vi "image.vi"(0 "Camera in":refnum<class "Camera.lvclass">, 5 "data_format":T2(ring)=enum."Mono16", 7 "image_index":u32, 9 "roi":cluster{"x0":u64, "y0":u64, "x1":u64, "y1":u64}={"x0"=18446744073709551615, "y0"=18446744073709551615, "x1"=18446744073709551615, "y1"=18446744073709551615}, 11 "error in (no error)":errorcluster, 12 "PCO_Recorder_CompressionParams":T5={"dGainK"=nan, "dDarkNoise_e"=nan, "dDSNU_e"=nan, "dPRNU_pct"=nan, "dLightSourceNoise_pct"=0.0}) -> (2 "timestamp":T4 {"lvTimestamp" format="%<%.6X\n%x>T"}, 3 "meta_data":T3, 4 "Camera out":refnum<class "Camera.lvclass">, 6 "image (U8)":u8[][](array[numeric]), 8 "image (U32)":u32[][](array[numeric]), 10 "image (U64)":T1(array[cluster]), 14 "raw_image (U16)":u16[][](array[numeric]), 15 "error out":errorcluster)   [LabVIEW 2019, in "Camera.lvclass"]
doc: "Get an image from the recorder. The type of the image is 2D array of pixel values. This array is\nshaped depending on the resolution and ROI of the image."
uses:
  Camera.lvclass
  pco.recorder/Recorder.lvlib
  pco.convert/Convert.lvlib
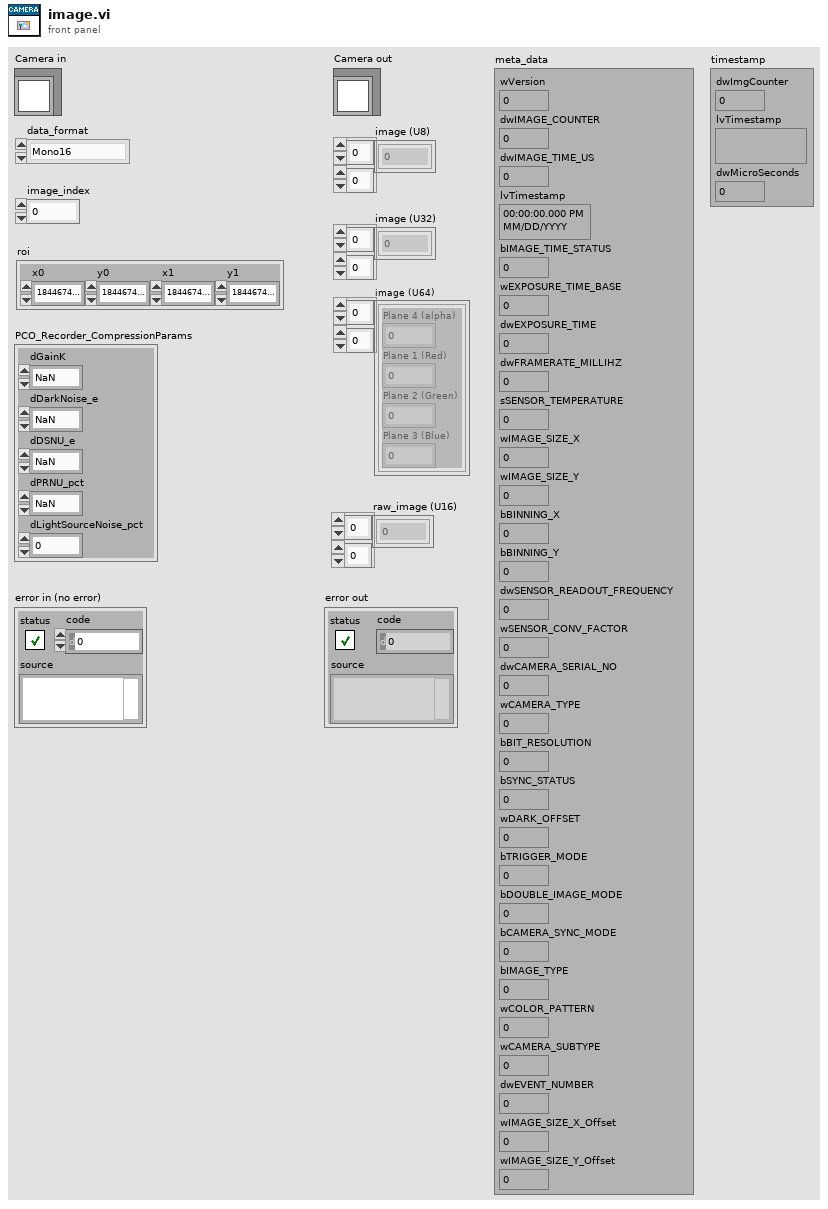
[diagram p1: front panel]
types:
  T1 = cluster{"Plane 4 (alpha)":u16, "Plane 1 (Red)":u16, "Plane 2 (Green)":u16, "Plane 3 (Blue)":u16}[][]
  T2 = enum16{"Undefined", "Mono8", "Mono16", "BGRA8", "RGBA8", "BGRA16", "RGBA16", "CompressedMono8"}
  T3 = cluster{"wVersion":u16, "dwIMAGE_COUNTER":u32, "dwIMAGE_TIME_US":u32, "lvTimestamp":timestamp, "bIMAGE_TIME_STATUS":u8, "wEXPOSURE_TIME_BASE":u16, "dwEXPOSURE_TIME":u32, "dwFRAMERATE_MILLIHZ":u32, "sSENSOR_TEMPERATURE":i16, "wIMAGE_SIZE_X":u16, "wIMAGE_SIZE_Y":u16, "bBINNING_X":u8, "bBINNING_Y":u8, "dwSENSOR_READOUT_FREQUENCY":u32, "wSENSOR_CONV_FACTOR":u16, "dwCAMERA_SERIAL_NO":u32, "wCAMERA_TYPE":u16, "bBIT_RESOLUTION":u8, "bSYNC_STATUS":u8, "wDARK_OFFSET":u16, "bTRIGGER_MODE":u8, "bDOUBLE_IMAGE_MODE":u8, "bCAMERA_SYNC_MODE":u8, "bIMAGE_TYPE":u8, "wCOLOR_PATTERN":u16, "wCAMERA_SUBTYPE":u16, "dwEVENT_NUMBER":u32, "wIMAGE_SIZE_X_Offset":u16, "wIMAGE_SIZE_Y_Offset":u16}
  T4 = cluster{"dwImgCounter":u32, "lvTimestamp":timestamp, "dwMicroSeconds":u32}
  T5 = cluster{"dGainK":dbl, "dDarkNoise_e":dbl, "dDSNU_e":dbl, "dPRNU_pct":dbl, "dLightSourceNoise_pct":dbl}
  T6 = map{enum16{"Undefined", "Mono8", "Mono16", "BGRA8", "RGBA8", "BGRA16", "RGBA16", "CompressedMono8"}, cluster{"sharpen":bool, "adaptive_sharpen":bool, "flip_vertical":bool, "auto_minmax":bool, "min_limit":u16, "max_limit":u16, "gamma":dbl, "contrast":i32, "pco_debayer_algorithm":bool, "color_temperature":i32, "color_saturation":i32, "color_vibrance":i32, "color_tint":i32, "lut_file":path}}
  T7 = map{enum16{"Undefined", "Mono8", "Mono16", "BGRA8", "RGBA8", "BGRA16", "RGBA16", "CompressedMono8"}, bool}
  T8 = cluster{"sharpen":bool, "adaptive_sharpen":bool, "flip_vertical":bool, "auto_minmax":bool, "min_limit":u16, "max_limit":u16, "gamma":dbl, "contrast":i32, "pco_debayer_algorithm":bool, "color_temperature":i32, "color_saturation":i32, "color_vibrance":i32, "color_tint":i32, "lut_file":path}
  T9 = map{enum16{"Undefined", "Mono8", "Mono16", "BGRA8", "RGBA8", "BGRA16", "RGBA16", "CompressedMono8"}, u64}
  T10 = cluster{"Blue":u16, "Green":u16, "Red":u16, "Alpha":u16}[][]
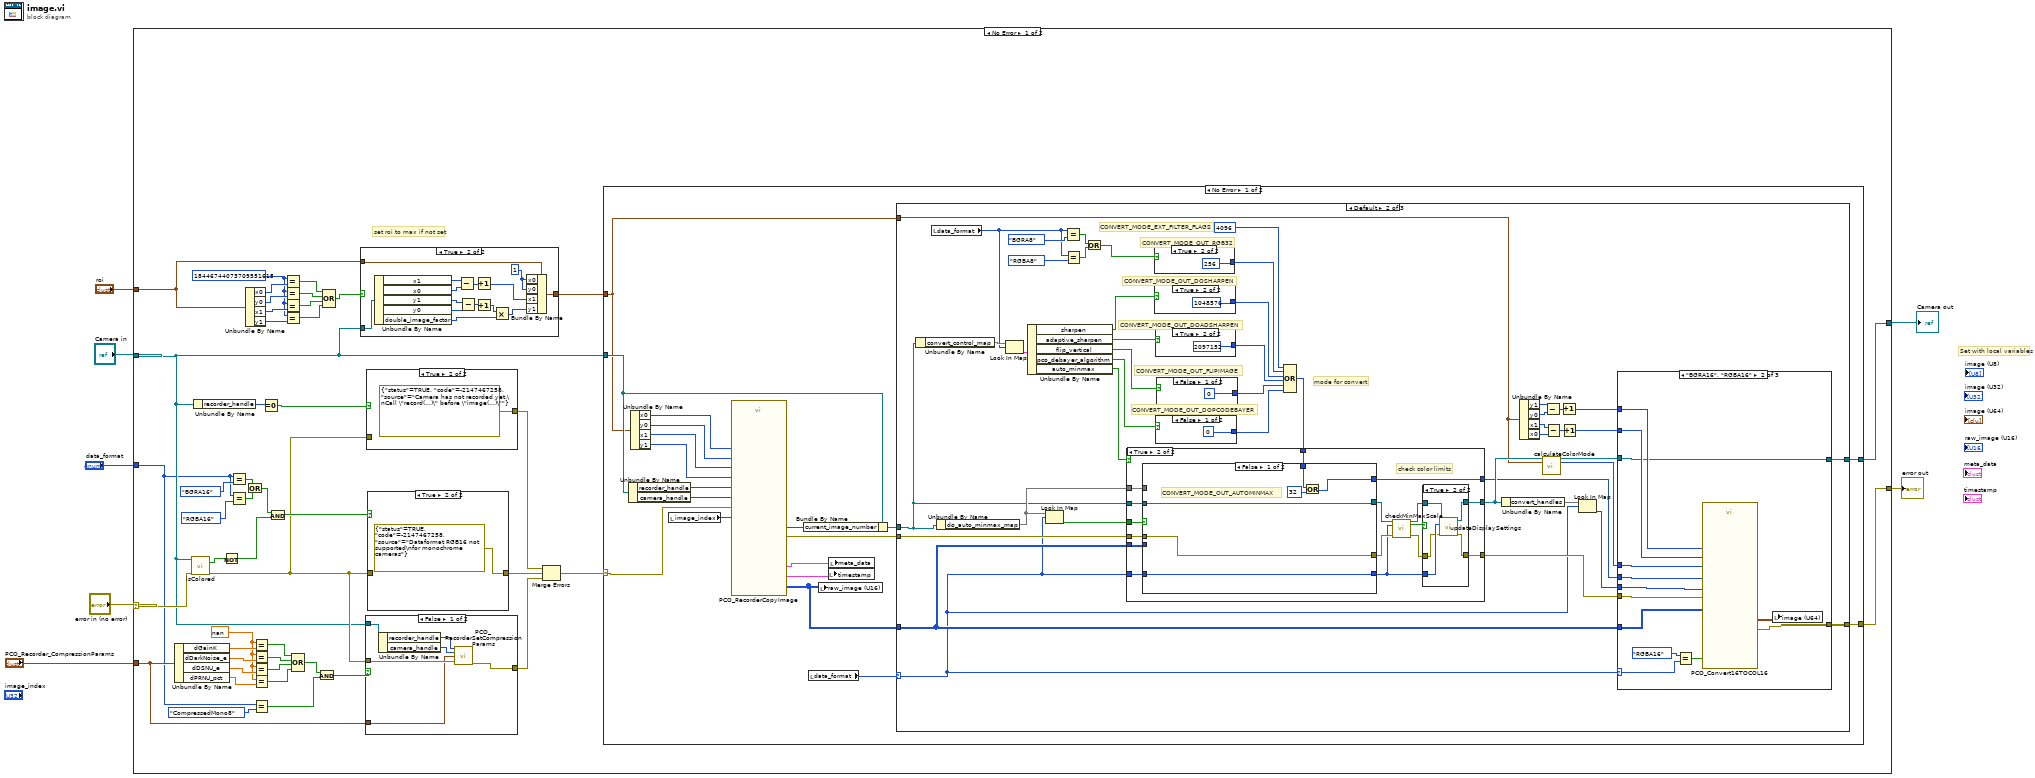
[diagram p0: block diagram]
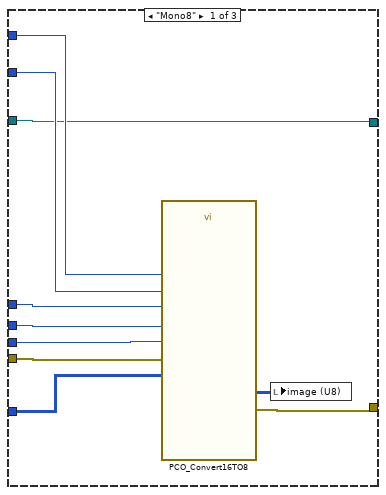
[diagram p4: hidden frame]
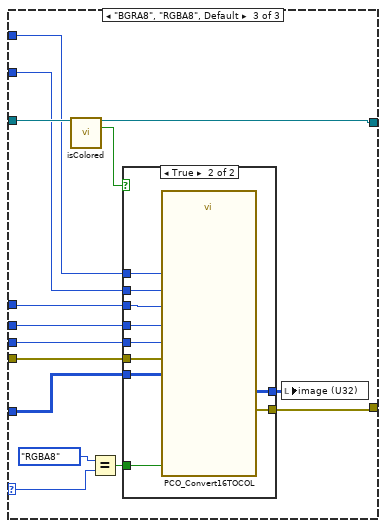
[diagram p5: hidden frame]
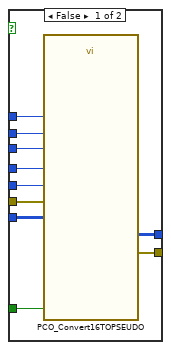
[diagram p6: hidden frame]
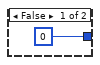
[diagram p7: hidden frame]
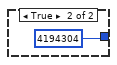
[diagram p8: hidden frame]
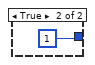
[diagram p9: hidden frame]
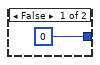
[diagram p10: hidden frame]
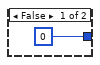
[diagram p11: hidden frame]
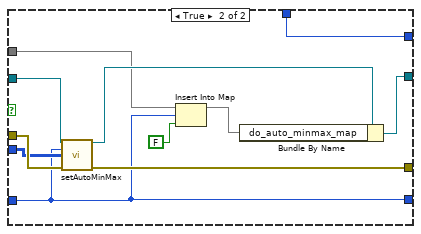
[diagram p14: hidden frame]
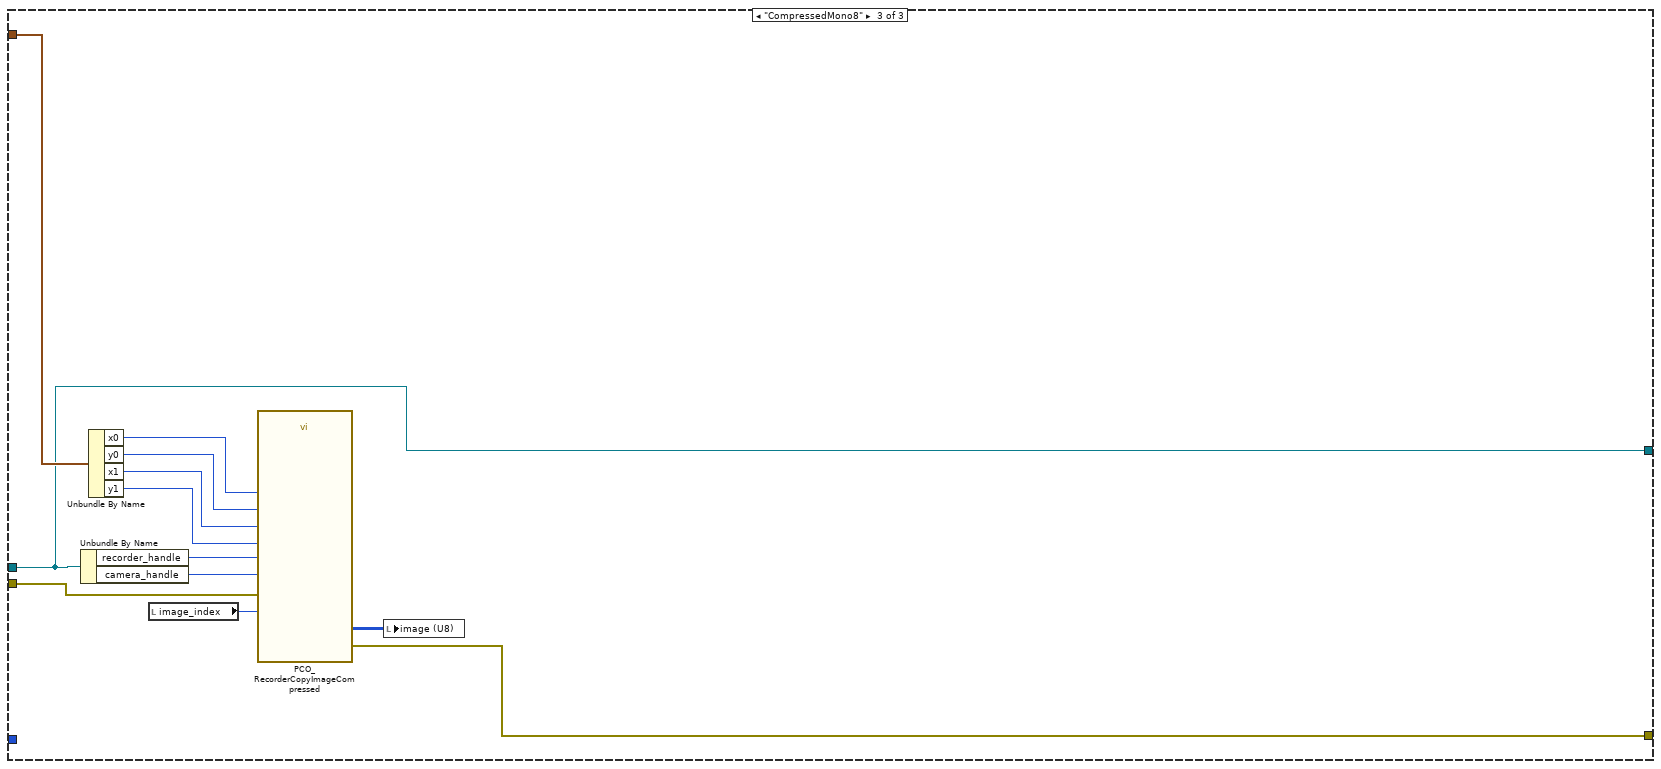
[diagram p15: hidden frame]
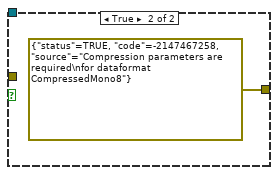
[diagram p19: hidden frame]
diagram:
  # "Set with local variables"
  n1 = case shown="No Error" "error in (no error)" {
    selector: "error in (no error)" -> [w53 w271]
    tunnel: [w19 w271] -> w6
    tunnel: [w20 w270] -> w4
    tunnel: "Camera in" -> [w16 w270]
    tunnel: "data_format" -> [w12 _]
    tunnel: "PCO_Recorder_CompressionParams" -> [w21 _]
    tunnel: "roi" -> [w17 _]
    frame No Error {
      w23 = u64 18446744073709551615 ("x0")
      w43 = nan ("dGainK")
      # "set roi to max if not set"
      n2 = Unbundle By Name(w21) -> ("dGainK"=w47:dbl, "dDarkNoise_e"=w46:dbl, "dDSNU_e"=w45:dbl, "dPRNU_pct"=w44:dbl)
      n3 = call-dynamic "isColored.vi"("Camera in"=w16, "error in (no error)"=w53) -> ("colored"=w52:bool, "error out"=w35:errorcluster)  [unwired: 11 in, 1 out]
      n4 = Unbundle By Name(w16) -> ("recorder_handle"=w49:u64)
      n5 = Not(x=w52) -> (.not. x?=w51:bool)
      n6 = Equal?(x=w12, y=T2."BGRA16" ("data_format")) -> (x = y?=w11:bool)
      n7 = Equal?(x=w12, y=T2."RGBA16" ("data_format")) -> (x = y?=w10:bool)
      n8 = Unbundle By Name(w17) -> ("x0"=w27:u64, "y0"=w26:u64, "x1"=w25:u64, "y1"=w24:u64)
      n9 = Or(x=w11, y=w10) -> (x .or. y?=w9:bool)
      n10 = Equal?(x=w43, y=w47) -> (x = y?=w42:bool)
      n11 = Equal?(x=w43, y=w46) -> (x = y?=w41:bool)
      n12 = Equal?(x=w43, y=w45) -> (x = y?=w40:bool)
      n13 = Equal?(x=w43, y=w44) -> (x = y?=w39:bool)
      n14 = Equal?(x=w12, y=T2."CompressedMono8" ("data_format")) -> (x = y?=w37:bool)
      n15 = Equal To 0?(x=w49) -> (x = 0?=w48:bool)
      n16 = And(x=w9, y=w51) -> (x .and. y?=w50:bool)
      n17 = Equal?(x=w23, y=w27) -> (x = y?=w28:bool)
      n18 = Equal?(x=w23, y=w26) -> (x = y?=w29:bool)
      n19 = Equal?(x=w23, y=w25) -> (x = y?=w30:bool)
      n20 = Equal?(x=w23, y=w24) -> (x = y?=w31:bool)
      n21 = Compound Arithmetic op=OR(w42, w41, w40, w39) -> (w38:bool)
      n22 = And(x=w38, y=w37) -> (x .and. y?=w36:bool)
      n23 = Compound Arithmetic op=OR(w28, w29, w30, w31) -> (w18:bool)
      n24 = case shown="True" w18 {
        tunnel: w16 -> [_ w68]
        tunnel: w17 -> [w54 w67]
        tunnel: [w54 w66] -> w15
        frame False {
        }
        frame True {
          w65 = u16 1 ("x0")
          n25 = Unbundle By Name(w68) -> ("x1"=w64:u64, "x0"=w63:u64, "y1"=w61:u64, "y0"=w60:u64, "double_image_factor"=w56:u16)
          n26 = Subtract(x=w64, y=w63) -> (x-y=w62:u64)
          n27 = Subtract(x=w61, y=w60) -> (x-y=w58:u64)
          n28 = Increment(x=w62) -> (x+1=w59:u64)
          n29 = Increment(x=w58) -> (x+1=w57:u64)
          n30 = Multiply(x=w57, y=w56) -> (x*y=w55:u64)
          n31 = Bundle By Name(cluster=w67, "x0"=w65, "y0"=w65, "x1"=w59, "y1"=w55) -> (w66:cluster{"x0":u64, "y0":u64, "x1":u64, "y1":u64})
        }
      }
      n32 = case shown="False" w36 {
        tunnel: [w263 errorcluster {"status"=TRUE, "code"=-2147467258, "source"="Compression parameters are required\nfor dataformat CompressedMono8"} ("error constant")] -> w32
        tunnel: w35 -> [w268 _]
        tunnel: w21 -> [w264 _]
        tunnel: w16 -> [w267 _]
        frame False {
          n33 = Unbundle By Name(w267) -> ("recorder_handle"=w266:u64, "camera_handle"=w265:u64)
          n34 = call "PCO_RecorderSetCompressionParams.vi"("phRec"=w266, "phCam"=w265, "strCompressionParams"=w264, "error in (no error)"=w268) -> ("error out"=w263:errorcluster)  [unwired: 9 in, 2 out]
        }
        frame True {
        }
      }
      n35 = case shown="True" w48 {
        tunnel: w35 -> [w259 _]
        tunnel: [w259 errorcluster {"status"=TRUE, "code"=-2147467258, "source"="Camera has not recorded yet.\nCall \"record(...)\" before \"image(...)\""} ("error constant")] -> w34
        frame False {
        }
        frame True {
        }
      }
      n36 = case shown="True" w50 {
        tunnel: w35 -> [w261 _]
        tunnel: [w261 errorcluster {"status"=TRUE, "code"=-2147467258, "source"="Dataformat RGB16 not supported\nfor monochrome cameras"} ("error constant")] -> w33
        frame False {
        }
        frame True {
        }
      }
      n37 = Merge Errors(w34, w33, w32) -> (w22:errorcluster)
      n38 = case shown="No Error" w22 {
        selector: w22 -> [w77 w258]
        tunnel: w15 -> [w71 _]
        tunnel: w16 -> [w76 w257]
        tunnel: [w70 w257] -> w20
        tunnel: [w69 w258] -> w19
        frame No Error {
          n39 = Unbundle By Name(w76) -> ("recorder_handle"=w82:u64, "camera_handle"=w83:u64)
          n40 = Unbundle By Name(w71) -> ("x0"=w78:u64, "y0"=w79:u64, "x1"=w80:u64, "y1"=w81:u64)
          n41 = local read "image_index"() -> (w84:u32)
          n42 = call "PCO_RecorderCopyImage.vi"("phRec"=w82, "phCam"=w83, "dwImgIdx"=w84, "wRoiX0"=w78, "wRoiY0"=w79, "wRoiX1"=w80, "wRoiY1"=w81, "error in (no error)"=w77) -> ("strTimestamp"=w85:T4, "strMetadata"=w86:T3, "wImgBuf"=w75:u16[][], "dwImgNumber"=w87:u32, "error out"=w74:errorcluster)  [unwired: 13 in, 2 out]
          n43 = Bundle By Name(cluster=w76, "current_image_number"=w87) -> (w73:refnum<class "Camera.lvclass">)
          n44 = local read "data_format"() -> (w72:T2)
          n45 = local write "raw_image (U16)"(w75) -> ()
          n46 = local write "timestamp"(w85) -> ()
          n47 = local write "meta_data"(w86) -> ()
          n48 = case shown="Default" w72 {
            selector: w72 -> [_ w90 _]
            tunnel: w74 -> [w88 w133 w249]
            tunnel: w75 -> [_ w120 _]
            tunnel: w73 -> [w89 w110 w246]
            tunnel: w71 -> [_ w130 w248]
            tunnel: [w89 w115 w246] -> w70
            tunnel: [w88 w114 w245] -> w69
            frame "Mono16" {
            }
            frame Default {
              # "CONVERT_MODE_OUT_RGB32"
              # "CONVERT_MODE_OUT_FLIPIMAGE"
              # "CONVERT_MODE_OUT_DOPCODEBAYER"
              # "CONVERT_MODE_OUT_DOADSHARPEN"
              # "CONVERT_MODE_OUT_DOSHARPEN"
              # "CONVERT_MODE_EXT_FILTER_FLAGS"
              # "mode for convert"
              n49 = Unbundle By Name(w110) -> ("convert_control_map"=w109:T6)
              n50 = local read "data_format"() -> (w95:T2)
              n51 = Unbundle By Name(w110) -> ("do_auto_minmax_map"=w112:T7)
              n52 = Look In Map(map=w109, key=w95) -> (value=w108:T8)  [unwired: 1 in, 1 out]
              n53 = Unbundle By Name(w108) -> ("sharpen"=w106:bool, "adaptive_sharpen"=w105:bool, "flip_vertical"=w97:bool, "pco_debayer_algorithm"=w104:bool, "auto_minmax"=w107:bool)
              n54 = Look In Map(map=w112, key=w90) -> (value=w113:bool)  [unwired: 1 in, 1 out]
              n55 = Equal?(x=w95, y=T2."BGRA8" ("data_format")) -> (x = y?=w93:bool)
              n56 = Equal?(x=w95, y=T2."RGBA8" ("data_format")) -> (x = y?=w92:bool)
              n57 = Or(x=w93, y=w92) -> (x .or. y?=w91:bool)
              n58 = case shown="True" w91 {
                tunnel: [u32 0 ("image_index") u32 256 ("image_index")] -> w98
                frame False {
                }
                frame True {
                }
              }
              n59 = case shown="True" w106 {
                tunnel: [u32 0 ("image_index") u32 1048576 ("image_index")] -> w103
                frame False {
                }
                frame True {
                }
              }
              n60 = case shown="True" w105 {
                tunnel: [u32 0 ("image_index") u32 2097152 ("image_index")] -> w102
                frame False {
                }
                frame True {
                }
              }
              n61 = case shown="False" w104 {
                tunnel: [u32 0 ("image_index") u32 4194304 ("image_index")] -> w100
                frame False {
                }
                frame True {
                }
              }
              n62 = case shown="False" w97 {
                tunnel: [u32 0 ("image_index") u32 1 ("image_index")] -> w101
                frame False {
                }
                frame True {
                }
              }
              n63 = Compound Arithmetic op=OR(u32 4096 ("image_index"), w98, w103, w102, w101, w100) -> (w111:u32)
              n64 = case shown="True" w107 {
                tunnel: w133 -> [w203 w220]
                tunnel: [w204 w207] -> w131
                tunnel: [w202 w219] -> w122
                tunnel: w120 -> [_ w218]
                tunnel: [w203 w206] -> w117
                tunnel: w113 -> [_ w217]
                tunnel: w112 -> [_ w216]
                tunnel: w111 -> [w202 w215]
                tunnel: w110 -> [w204 w214]
                tunnel: w90 -> [_ w213]
                frame False {
                }
                frame True {
                  # "check color limits"
                  n65 = case shown="False" w217 {
                    tunnel: w214 -> [w229 w244]
                    tunnel: w215 -> [w231 w236]
                    tunnel: [w230 w236] -> w219
                    tunnel: w218 -> [_ w235]
                    tunnel: w213 -> [w228 w234]
                    tunnel: [w229 w243] -> w212
                    tunnel: w220 -> [w233 w242]
                    tunnel: [w233 w241] -> w211
                    tunnel: w216 -> [_ w237]
                    tunnel: [w228 w234] -> w205
                    frame False {
                      # "CONVERT_MODE_OUT_AUTOMINMAX"
                      n66 = Or(x=w231, y=u32 32 ("image_index")) -> (x .or. y?=w230:u32)
                    }
                    frame True {
                      n67 = call-dynamic "setAutoMinMax.vi"("Camera in"=w244, "data_format"=w234, "image"=w235, "error in (no error)"=w242) -> ("Camera out"=w239:refnum<class "Camera.lvclass">, "error out"=w241:errorcluster)  [unwired: 10 in]
                      n68 = Insert Into Map(map in=w237, key=w234, value=FALSE) -> (map out=w238:T7)  [unwired: 2 out]
                      n69 = Bundle By Name(cluster=w239, "do_auto_minmax_map"=w238) -> (w243:refnum<class "Camera.lvclass">)
                    }
                  }
                  n70 = call-dynamic "checkMinMaxScale.vi"("Camera in"=w212, "data_format"=w205, "error in (no error)"=w211) -> ("Camera out"=w209:refnum<class "Camera.lvclass">, "needsUpdate"=w210:bool, "error out"=w208:errorcluster)  [unwired: 10 in]
                  n71 = case shown="True" w210 {
                    tunnel: w209 -> [w222 w227]
                    tunnel: w208 -> [w221 w223]
                    tunnel: [w222 w225] -> w207
                    tunnel: [w221 w226] -> w206
                    tunnel: w205 -> [_ w224]
                    frame False {
                    }
                    frame True {
                      n72 = call-dynamic "updateDisplaySettings.vi"("Camera in"=w227, "data_format"=w224, "error in (no error)"=w223) -> ("Camera out"=w225:refnum<class "Camera.lvclass">, "error out"=w226:errorcluster)  [unwired: 11 in]
                    }
                  }
                }
              }
              n73 = Unbundle By Name(w131) -> ("convert_handles"=w132:T9)
              n74 = Unbundle By Name(w130) -> ("y1"=w128:u64, "y0"=w129:u64, "x1"=w127:u64, "x0"=w126:u64)
              n75 = call-dynamic "calculateColorMode.vi"("Camera in"=w131, "roi"=w130) -> ("Camera out"=w116:refnum<class "Camera.lvclass">, "colorMode"=w121:i32)  [unwired: 11 in, 1 out]
              n76 = Subtract(x=w128, y=w129) -> (x-y=w125:u64)
              n77 = Subtract(x=w127, y=w126) -> (x-y=w124:u64)
              n78 = Increment(x=w125) -> (x+1=w119:u64)
              n79 = Increment(x=w124) -> (x+1=w118:u64)
              n80 = Look In Map(map=w132, key=w90) -> (value=w123:u64)  [unwired: 1 in, 1 out]
              n81 = case shown="\"BGRA16\", \"RGBA16\"" w90 {
                selector: w90 -> [_ w146 w158]
                tunnel: w123 -> [w138 w151 w164]
                tunnel: w122 -> [w139 w152 w161]
                tunnel: w121 -> [w140 w153 w160]
                tunnel: w120 -> [w136 w154 w170]
                tunnel: w119 -> [w142 w156 w163]
                tunnel: w118 -> [w141 w155 w162]
                tunnel: w117 -> [w137 w150 w165]
                tunnel: w116 -> [w134 w148 w169]
                tunnel: [w134 w148 w167] -> w115
                tunnel: [w135 w149 w168] -> w114
                frame "Mono8" {
                  n82 = call "PCO_Convert16TO8.vi"("ph"=w138, "height"=w142, "mode"=w139, "icolmode"=w140, "width"=w141, "error in (no error)"=w137, "b16"=w136) -> ("b8"=w143:u8[][], "error out"=w135:errorcluster)  [unwired: 5 in, 2 out]
                  n83 = local write "image (U8)"(w143) -> ()
                }
                frame "BGRA16", "RGBA16" {
                  n84 = Equal?(x=T2."RGBA16" ("data_format"), y=w146) -> (x = y?=w145:bool)
                  n85 = call "PCO_Convert16TOCOL16.vi"("ph"=w151, "height"=w156, "swap_colors"=w145, "mode"=w152, "icolmode"=w153, "width"=w155, "error in (no error)"=w150, "raw_image(U16)"=w154) -> ("image (U64)"=w144:T10, "error out"=w149:errorcluster)  [unwired: 4 in, 2 out]
                  n86 = local write "image (U64)"(w144) -> ()
                }
                frame "BGRA8", "RGBA8", Default {
                  n87 = call-dynamic "isColored.vi"("Camera in"=w169) -> ("Camera out"=w167:refnum<class "Camera.lvclass">, "colored"=w171:bool)  [unwired: 12 in, 1 out]
                  n88 = Equal?(x=T2."RGBA8" ("data_format"), y=w158) -> (x = y?=w157:bool)
                  n89 = case shown="True" w171 {
                    tunnel: w170 -> [w179 w190]
                    tunnel: [w181 w191] -> w168
                    tunnel: [w180 w183] -> w166
                    tunnel: w165 -> [w178 w189]
                    tunnel: w164 -> [w177 w188]
                    tunnel: w163 -> [w173 w187]
                    tunnel: w162 -> [w174 w186]
                    tunnel: w161 -> [w176 w185]
                    tunnel: w160 -> [w175 w182]
                    tunnel: w157 -> [w172 w184]
                    frame False {
                      n90 = call "PCO_Convert16TOPSEUDO.vi"("ph"=w177, "height"=w173, "swap_colors"=w172, "mode"=w176, "icolmode"=w175, "width"=w174, "error in (no error)"=w178, "b16"=w179) -> ("b32"=w180:u32[][], "error out"=w181:errorcluster)  [unwired: 4 in, 2 out]
                    }
                    frame True {
                      n91 = call "PCO_Convert16TOCOL.vi"("ph"=w188, "height"=w187, "swap_colors"=w184, "mode"=w185, "icolmode"=w182, "width"=w186, "error in (no error)"=w189, "b16"=w190) -> ("b32"=w183:u32[][], "error out"=w191:errorcluster)  [unwired: 4 in, 2 out]
                    }
                  }
                  n92 = local write "image (U32)"(w166) -> ()
                }
              }
            }
            frame "CompressedMono8" {
              n93 = Unbundle By Name(w246) -> ("recorder_handle"=w252:u64, "camera_handle"=w251:u64)
              n94 = Unbundle By Name(w248) -> ("x0"=w256:u64, "y0"=w255:u64, "x1"=w254:u64, "y1"=w253:u64)
              n95 = local read "image_index"() -> (w250:u32)
              n96 = call "PCO_RecorderCopyImageCompressed.vi"("phRec"=w252, "phCam"=w251, "dwImgIdx"=w250, "wRoiX0"=w256, "wRoiY0"=w255, "wRoiX1"=w254, "wRoiY1"=w253, "error in (no error)"=w249) -> ("bImgBuf"=w247:u8[][], "error out"=w245:errorcluster)  [unwired: 13 in, 5 out]
              n97 = local write "image (U8)"(w247) -> ()
            }
          }
        }
        frame Error {
        }
      }
    }
    frame Error {
    }
  }
  "error out" <- w6
  "Camera out" <- w4
